vi "Product Selected USD.vi"(8 "error in (no error)":errorcluster, 10 "Product Selected":i32, 11 "USD Actor in":refnum<class "USD Actor.lvclass">) -> (0 "error out":errorcluster, 3 "USD Actor out":refnum<class "USD Actor.lvclass">)   [LabVIEW 2020, in "USD Actor.lvlib" / "USD Actor.lvclass"]
uses:
  USD Actor.lvclass
  USD Actor.lvclass/USD Actor.ctl
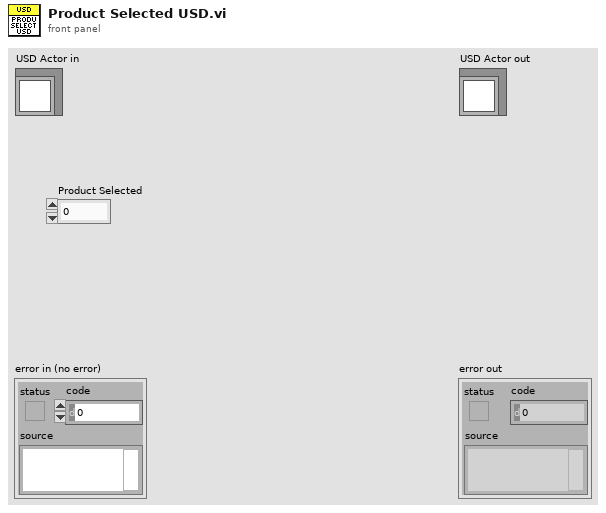
[diagram p1: front panel]
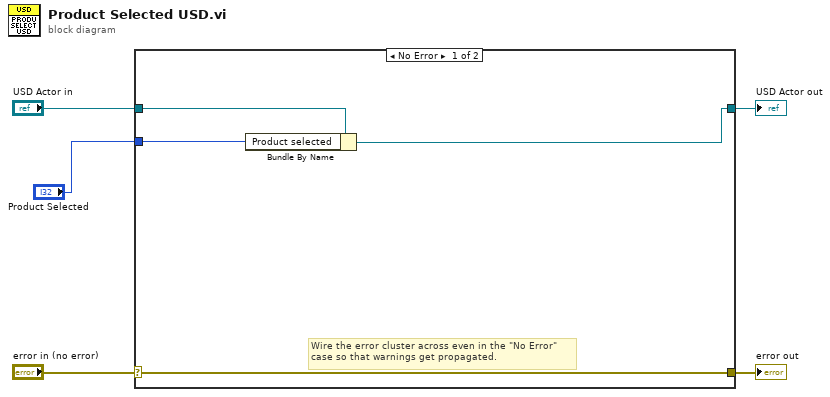
[diagram p0: block diagram]
diagram:
  n1 = case shown="No Error" "error in (no error)" {
    selector: "error in (no error)" -> [w9 w11]
    tunnel: [w9 w11] -> w4
    tunnel: [w7 w10] -> w2
    tunnel: "USD Actor in" -> [w8 w10]
    tunnel: "Product Selected" -> [w6 _]
    frame No Error {
      # "Wire the error cluster across even in the \"No Error\"\ncase so that warnings get propagated."
      n2 = Bundle By Name(cluster=w8, "Product selected"=w6) -> (w7:refnum<class "USD Actor.lvclass">)
    }
    frame Error {
    }
  }
  "error out" <- w4
  "USD Actor out" <- w2
